vi "2dsmooth (SubVI).vi"(8 "Filter order (2)":i32=2 min=1 max=1000 step=1, 9 "Cutoff frq (0.125)":dbl=0.125, 11 "Data":sgl[][](array[numeric])) -> (3 "Y out":dbl[][](array[numeric]))   [LabVIEW 2014]
uses:
  <userlib>/Nanonis Prog Interface V5/Nanonis Prog Interface.lvlib
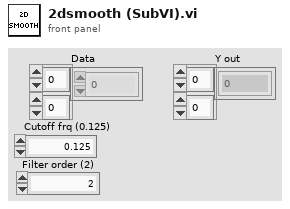
[diagram p1: front panel]
types:
  T1 = enum16{"none", "Gaussian", "Butterworth", "5th order FIR"}
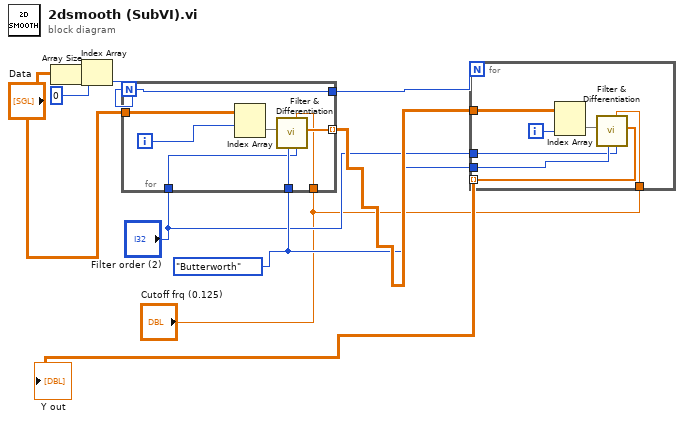
[diagram p0: block diagram]
diagram:
  w3 = T1."Butterworth" ("Filter type (none)")
  n1 = Array Size(array="Data") -> (size(s)=w7:i32[])
  n2 = Index Array(array=w7, index=0) -> (element=w8:i32)
  n3 = for {
    N: w8 -> [w14]
    tunnel: "Data" -> [w18]
    tunnel: [w15] -> w4 mode=indexing
    tunnel: [w14] -> w10
    tunnel: w3 -> [w13]
    tunnel: "Cutoff frq (0.125)" -> [w12]
    tunnel: "Filter order (2)" -> [w11]
    i -> [w16]
    n4 = Index Array(array=w18, index (row)=w16) -> (element=w17:sgl[])  [unwired: 1 in]
    n5 = call <userlib>:"Filter & Differentiation.vi"("Filter order (2)"=w11, "Cutoff frq (0.125)"=w12, "Filter type (none)"=w13, "Y in"=w17) -> ("Y out"=w15:dbl[])  [unwired: 5 in, 2 out]
  }
  n6 = for {
    N: w10 -> [_]
    tunnel: w4 -> [w25]
    tunnel: [w22] -> w5 mode=indexing
    tunnel: w3 -> [w21]
    tunnel: "Filter order (2)" -> [w20]
    tunnel: "Cutoff frq (0.125)" -> [w19]
    i -> [w23]
    n7 = Index Array(array=w25, index (col)=w23) -> (element=w24:dbl[])  [unwired: 1 in]
    n8 = call <userlib>:"Filter & Differentiation.vi"("Filter order (2)"=w20, "Cutoff frq (0.125)"=w19, "Filter type (none)"=w21, "Y in"=w24) -> ("Y out"=w22:dbl[])  [unwired: 5 in, 2 out]
  }
  "Y out" <- w5
